vi "CoboltLaser_ModeSet.vi"(0 "ComPort":refnum<visa-resource-name>, 5 "Mode":T1 caption="Laser Mode", 7 "CheckResponse":bool=TRUE, 11 "ErrorIn":errorcluster) -> (4 "ComPortOut":refnum<visa-resource-name>, 8 "Response":string, 10 "Units(mA:1)":bool, 15 "ErrorOut":errorcluster)   [LabVIEW 2019]
doc: "Use this template to build a VI to use as a subVI."
uses:
  Programmes Labview/LabScanV1A/DevicesClass/InstrumentsClass/CoboltMLD/CoboltModes.ctl
panel:
  out "ResponseOK":bool
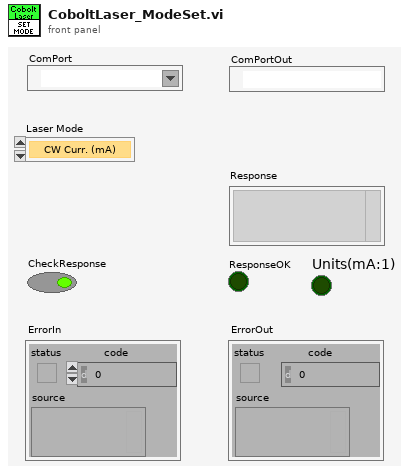
[diagram p1: front panel]
types:
  T1 = typedef "CoboltModes.ctl" = enum16{"CW Curr. (mA)", "CW Pow. (mW)", "Curr. Mod. (mA)", "Pow. Mod. (mW)"}
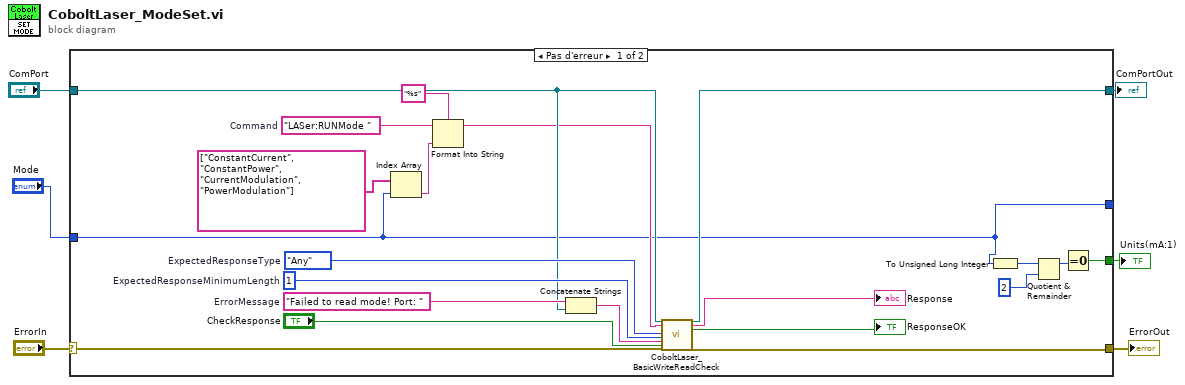
[diagram p0: block diagram]
diagram:
  n1 = case shown="Pas d'erreur" "ErrorIn" {
    selector: "ErrorIn" -> [w27 w29]
    tunnel: [w26 w29] -> w5
    tunnel: "ComPort" -> [w19 w28]
    tunnel: [w18 w28] -> w3
    tunnel: [w9 _] -> _
    tunnel: [w12 _] -> w2
    tunnel: "Mode" -> [w9 _]
    frame No Error {
      w24 = 1  # ExpectedResponseMinimumLength
      w25 = enum16{"Any", "Digits Only", "Non-Digits Only"}."Any"  # ExpectedResponseType
      w21 = "Failed to read mode! Port: "  # ErrorMessage
      w17 = "LASer:RUNMode "  # Command
      n2 = Index Array(array=string[] ["ConstantCurrent", "ConstantPower", "CurrentModulation", "PowerModulation"], index=w9) -> (element=w7:string)
      n3 = Format Into String(format string="%s" ("chaîne de format"), initial string=w17, w7) -> (resulting string=w11:string)  [unwired: 1 in, 1 out]
      n4 = Concatenate Strings(w21, w19) -> (w20:string)
      n5 = call <userlib>:"CoboltLaser_BasicWriteReadCheck.vi"("ComPort"=w19, "Command"=w11, "ExpectedResponseType"=w25, "ExpectedResponseMinimumLength"=w24, "ErrorMessage"=w20, "GenerateError"="CheckResponse", "error in (no error)"=w27) -> ("ComPortOut"=w18:refnum<visa-resource-name>, "Response"=→"Response":string, "ResponseOK"=→"ResponseOK":bool, "error out"=w26:errorcluster)  [unwired: 17 in]
      n6 = To Unsigned Long Integer(number=w9) -> (unsigned 32bit integer=w15:u32)
      n7 = Quotient & Remainder(x=w15, y=u32 2) -> (x-y*floor(x/y)=w13:u32)  [unwired: 1 out]
      n8 = Equal To 0?(x=w13) -> (x = 0?=w12:bool)
    }
    frame Error {
    }
  }
  "ErrorOut" <- w5
  "ComPortOut" <- w3
  "Units(mA:1)" <- w2
